vi "Export DMA Channels RTM.vi"(8 "error in (no error)":errorcluster, 11 "Node Ptr":u64 format="%.0x") -> (0 "error out":errorcluster)   [LabVIEW 2019, in "FPGA Addon System Explorer.lvlib"]
uses:
  FPGA Addon System Explorer.lvlib
  <vilib>/NI VeriStand/Custom Device API/Custom Device Waveform DataType.ctl
  <vilib>/Utility/file.llb/Write Delimited Spreadsheet (string).vi
  <vilib>/NI VeriStand/Custom Device Tools/Custom Device Utility Library/Custom Device Utility Library.lvlib
  <vilib>/NI VeriStand/Custom Device API/Custom Device API.lvlib
panel:
  in  "Tag":string
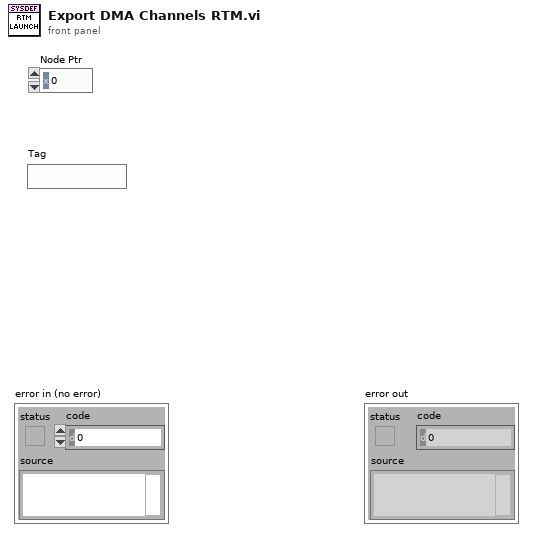
[diagram p1: front panel]
types:
  T1 = typedef "Custom Device API.lvlib/Custom Device Waveform DataType.ctl" = enum16{"Double", "Complex Double"}
  T2 = typedef "Custom Device API.lvlib/Custom Device Item Ref.ctl" = u64
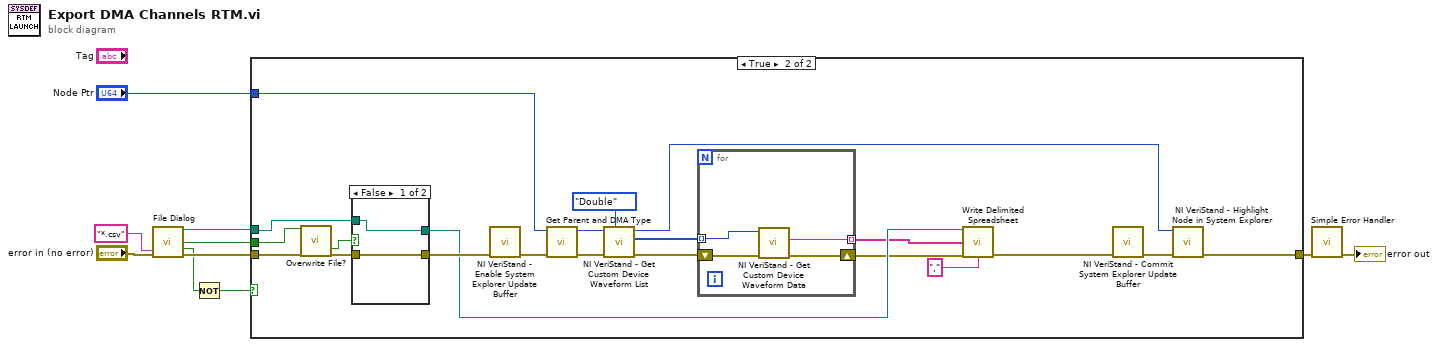
[diagram p0: block diagram]
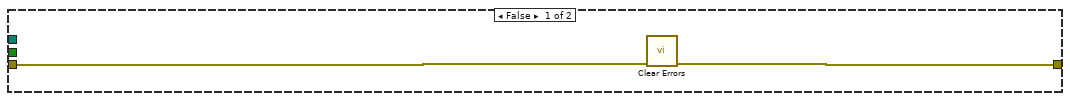
[diagram p2: hidden frame]
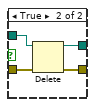
[diagram p3: hidden frame]
diagram:
  n1 = call "File Dialog"("error in"="error in (no error)", "pattern (all files)"="*.csv") -> ("selected path"=w9:path, "exists"=w1:bool, "cancelled"=w3:bool, "error out"=w8:errorcluster)  [unwired: 10 in]
  n2 = Not(x=w3) -> (.not. x?=w2:bool)
  n3 = case shown="True" w2 {
    tunnel: w9 -> [_ w25]
    tunnel: w8 -> [w12 w28]
    tunnel: "Node Ptr" -> [_ w33]
    tunnel: [w11 w30] -> w4
    tunnel: w1 -> [_ w29]
    frame False {
      n4 = call <vilib>:"Clear Errors.vi"("error in (no error)"=w12) -> ("error out"=w11:errorcluster)  [unwired: 5 in, 1 out]
    }
    frame True {
      n5 = call "Overwrite File?"("Enable"=w29, "error in (no error)"=w28) -> ("Yes"=w27:bool, "error out"=w26:errorcluster)  [unwired: 16 in]
      n6 = case shown="False" w27 {
        tunnel: w26 -> [w39 w43]
        tunnel: w25 -> [w38 w42]
        tunnel: [w39 w40] -> w24
        tunnel: [w38 w41] -> w23
        frame False {
        }
        frame True {
          n7 = Delete(path (use dialog)=w42, error in=w43) -> (deleted path=w41:path, error out=w40:errorcluster)  [unwired: 3 in, 1 out]
        }
      }
      n8 = call <vilib>:"NI VeriStand - Enable System Explorer Update Buffer.vi"("error in (no error)"=w24) -> ("error out"=w31:errorcluster)  [unwired: 10 in]
      n9 = call "Get Parent and DMA Type.vi"("error in (no error)"=w31, "Node Ptr"=w33) -> ("error out"=w18:errorcluster, "Item Ref out"=w20:T2)  [unwired: 6 in, 2 out]
      n10 = call <vilib>:"NI VeriStand - Get Custom Device Waveform List.vi"("Waveform Data Type"=Custom_Device_Waveform_DataType."Double", "error in (no error)"=w18, "Device Ref in"=w20) -> ("error out"=w15:errorcluster, "Specified Waveform Ref List"=w17:T2[], "Device Ref out"=w16:T2)  [unwired: 6 in]
      n11 = for {
        tunnel: w17 -> [w35] mode=indexing
        shift-right: [w36] -> w14
        shift-left: w15 -> [w37]
        tunnel: [w34] -> w13 mode=indexing
        n12 = call <vilib>:"NI VeriStand - Get Custom Device Waveform Data.vi"("error in (no error)"=w37, "Waveform Ref in"=w35) -> ("error out"=w36:errorcluster, "Waveform Name"=w34:string)  [unwired: 4 in, 4 out]
      }
      n13 = call-poly <vilib>:"Write Delimited Spreadsheet.vi"("file path (dialog if empty)"=w23, "1D data"=w13, "error in (no error)"=w14, "delimiter (\\t)"="," ("delimiter (\\t)")) -> ("error out"=w21:errorcluster)  [unwired: 10 in, 1 out]
      n14 = call <vilib>:"NI VeriStand - Commit System Explorer Update Buffer.vi"("error in (no error)"=w21) -> ("error out"=w32:errorcluster)  [unwired: 10 in]
      n15 = call <vilib>:"NI VeriStand - Highlight Node in System Explorer.vi"("error in (no error)"=w32, "Item Ref in"=w16) -> ("error out"=w30:errorcluster)  [unwired: 8 in, 1 out]
    }
  }
  n16 = call <vilib>:"Simple Error Handler.vi"("error in (no error)"=w4) -> ("error out"=→"error out":errorcluster)  [unwired: 4 in, 4 out]
